vi "Parse String.vi"(2 "String In":string) -> (0 "Array Out":string[](array[string]), 1 "Source":bool)   [LabVIEW 2013]
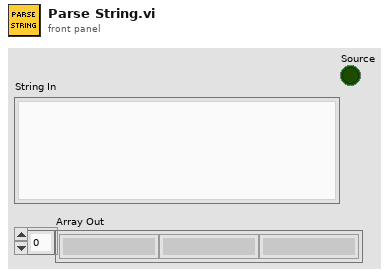
[diagram p1: front panel]
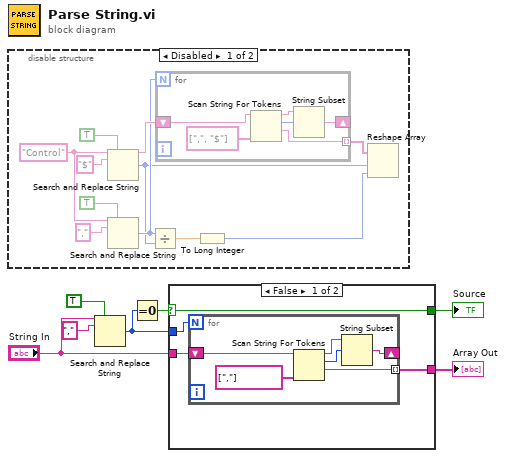
[diagram p0: block diagram]
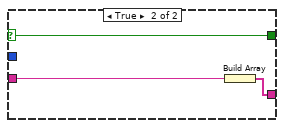
[diagram p2: hidden frame]
diagram:
  n1 = disable-structure shown="Disabled" {
    frame Disabled {
      w8 = "Control" ("input string")
      n2 = Search and Replace String(replace all?=TRUE ("replace all? (F)"), input string=w8, search string="$") -> (result string=w14:string, number of replacements=w10:i32)  [unwired: 5 in, 2 out]
      n3 = Search and Replace String(replace all?=TRUE ("replace all? (F)"), input string=w8, search string=",") -> (number of replacements=w13:i32)  [unwired: 5 in, 3 out]
      n4 = Divide(x=w13, y=w10) -> (x/y=w12:dbl)
      n5 = for {
        N: w13 -> [_]
        shift-right: [w20] -> _
        shift-left: w14 -> [w21]
        tunnel: [w19] -> w9 mode=indexing
        n6 = Scan String For Tokens(6:string[] [",", "$"] ("delimiters (\\s,\\t,\\r,\\n)"), 9:w21) -> (1:w19:string, 2:w23:i32, 3:w22:string)  [unwired: 4 in, 1 out]
        n7 = String Subset(string=w22, offset (0)=w23) -> (substring=w20:string)  [unwired: 1 in]
      }
      n8 = To Long Integer(number=w12) -> (32bit integer=w11:i32)
      n9 = Reshape Array(w9, w10, w11) -> ()  [unwired: 1 out]
    }
    frame Enabled {
    }
  }
  n10 = Search and Replace String(replace all?=TRUE ("replace all? (F)"), input string="String In", search string=",") -> (number of replacements=w4:i32)  [unwired: 5 in, 3 out]
  n11 = Equal To 0?(x=w4) -> (x = 0?=w3:bool)
  n12 = case shown="False" w3 {
    selector: w3 -> [w25 w35]
    tunnel: "String In" -> [w28 w36]
    tunnel: w4 -> [w27 _]
    tunnel: [w26 w37] -> w2
    tunnel: [w25 w35] -> w1
    frame False {
      n13 = for {
        N: w27 -> [_]
        tunnel: [w30] -> w26 mode=indexing
        shift-right: [w29] -> _
        shift-left: w28 -> [w34]
        n14 = Scan String For Tokens(6:string[] [","] ("delimiters (\\s,\\t,\\r,\\n)"), 9:w34) -> (1:w30:string, 2:w31:i32, 3:w32:string)  [unwired: 4 in, 1 out]
        n15 = String Subset(string=w32, offset (0)=w31) -> (substring=w29:string)  [unwired: 1 in]
      }
    }
    frame True {
      n16 = Build Array(w36) -> (w37:string[])
    }
  }
  "Array Out" <- w2
  "Source" <- w1
